vi "Create Loc String Object.vi"(10 "Error In":errorcluster, 11 "String Input":string) -> (2 "Error Out":errorcluster, 3 "Loc String .NET Ref":refnum<k24>)   [LabVIEW 2019, in "VeriStand Custom Device XML Parser.lvlib"]
doc: "Create a Loc string object based off the string input"
uses:
  VeriStand Custom Device XML Parser.lvlib
  NationalInstruments.VeriStand.XMLReader
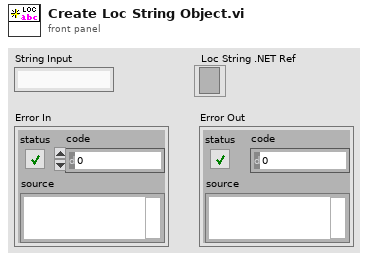
[diagram p1: front panel]
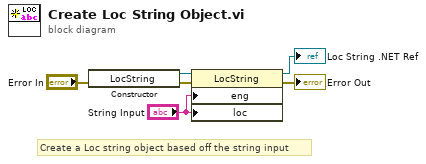
[diagram p0: block diagram]
diagram:
  # "Create a Loc string object based off the string input"
  n1 = constructor class="LocString"(error in="Error In") -> (reference out=w5:refnum<k24>, error out=w6:errorcluster)  [unwired: 2 in, 1 out]
  n2 = property class="LocString"(reference=w5, error in=w6, "eng"="String Input", "loc"="String Input") -> (reference out=→"Loc String .NET Ref":refnum<k24>, error out=→"Error Out":errorcluster)
